vi "Osciloskop.vi"() -> ()   [LabVIEW 2026]
uses:
  <vilib>/express/express analysis/Spectral/XNode/ExpressSpectralMeasurementsBlockNode.xnode
  <vilib>/express/express analysis/Spectral/Block/exnSpectralBlock spectral measurements RMS poly.vi
  <vilib>/express/express analysis/Spectral/Block/exnSpectralBlock spectral measurements RMS DDT.vi
  <instrlib>/niScope/Controls/niScope scalar measurement.ctl
  <instrlib>/niScope/Utility/niScope Get Channel Name From String.vi
  <instrlib>/niScope/Acquire/Fetch/niScope Fetch WDT.vi
  <vilib>/express/express analysis/Spectral/Block/exnSpectralBlock spectral measurements peak poly.vi
  <vilib>/express/express analysis/Spectral/Block/exnSpectralBlock spectral measurements peak DDT.vi
  <vilib>/express/express analysis/Spectral/Block/exnSpectralBlock spectral measurements power poly.vi
  <vilib>/express/express analysis/Spectral/Block/exnSpectralBlock spectral measurements power DDT.vi
  <vilib>/express/express analysis/Spectral/Block/exnSpectralBlock spectral measurements PSD poly.vi
  <vilib>/express/express analysis/Spectral/Block/exnSpectralBlock spectral measurements PSD DDT.vi
panel:
  out "FFT":dynamicdata(graph)
  out "Waveform Graph":waveform(dbl)[](graph)
  in  "Resource name":refnum<k15> caption="Uredjaj"
  in  "Start/Pauza":bool
  in  "Simulacija":bool
  in  "Measurement 5":T1=6 caption="Measurement 4" items=["None"=4000, "Frequency"=2, "Average Frequency"=1016, "FFT Frequency"=1008, "Period"=3, "Average Period"=1015, "Rise Time"=0, "Fall Time"=1, "Rising Slew Rate"=1010, "Falling Slew Rate"=1011, "Overshoot"=18, "Preshoot"=19, "Voltage RMS"=4, "Voltage Cycle RMS"=16, "AC Estimate"=1012, "FFT Amplitude"=1009, "Voltage Average"=10, "Voltage Cycle Average"=17, "DC Estimate"=1013, "Voltage Max"=6, "Voltage Min"=7, "Voltage Peak-to-Peak"=5, "Voltage High"=8, "Voltage Low"=9, "Voltage Amplitude"=15, "Voltage Top"=1007, "Voltage Base"=1006, "Voltage Base-to-Top"=1017, "Negative Width"=11, "Positive Width"=12, "Negative Duty Cycle"=13, "Positive Duty Cycle"=14, "Integral"=1005, "Area"=1003, "Cycle Area"=1004, "Time Delay"=1014, "Phase Delay"=1018, "Low Ref Volts"=1000, "Mid Ref Volts"=1001, "High Ref Volts"=1002, "Volt. Hist. Mean"=2000, "Volt. Hist. Stdev"=2001, "Volt. Hist. Median"=2003, "Volt. Hist. Mode"=2010, "Volt. Hist. Max"=2005, "Volt. Hist. Min"=2006, "Volt. Hist. Peak-to-Peak"=2002, "Volt. Hist. Mean + Stdev"=2007, "Volt. Hist. Mean + 2 Stdev"=2008, "Volt. Hist. Mean + 3 Stdev"=2009, "Volt. Hist. Hits"=2004, "Volt. Hist. New Hits"=2011, "Time Hist. Mean"=3000, "Time Hist. Stdev"=3001, "Time Hist. Median"=3003, "Time Hist. Mode"=3010, "Time Hist. Max"=3005, "Time Hist. Min"=3006, "Time Hist. Peak-to-Peak"=3002, "Time Hist. Mean + Stdev"=3007, "Time Hist. Mean + 2 Stdev"=3008, "Time Hist. Mean + 3 Stdev"=3009, "Time Hist. Hits"=3004, "Time Hist. New Hits"=3011]
  in  "Measurement 4":T1=5 caption="Measurement 3" items=["None"=4000, "Frequency"=2, "Average Frequency"=1016, "FFT Frequency"=1008, "Period"=3, "Average Period"=1015, "Rise Time"=0, "Fall Time"=1, "Rising Slew Rate"=1010, "Falling Slew Rate"=1011, "Overshoot"=18, "Preshoot"=19, "Voltage RMS"=4, "Voltage Cycle RMS"=16, "AC Estimate"=1012, "FFT Amplitude"=1009, "Voltage Average"=10, "Voltage Cycle Average"=17, "DC Estimate"=1013, "Voltage Max"=6, "Voltage Min"=7, "Voltage Peak-to-Peak"=5, "Voltage High"=8, "Voltage Low"=9, "Voltage Amplitude"=15, "Voltage Top"=1007, "Voltage Base"=1006, "Voltage Base-to-Top"=1017, "Negative Width"=11, "Positive Width"=12, "Negative Duty Cycle"=13, "Positive Duty Cycle"=14, "Integral"=1005, "Area"=1003, "Cycle Area"=1004, "Time Delay"=1014, "Phase Delay"=1018, "Low Ref Volts"=1000, "Mid Ref Volts"=1001, "High Ref Volts"=1002, "Volt. Hist. Mean"=2000, "Volt. Hist. Stdev"=2001, "Volt. Hist. Median"=2003, "Volt. Hist. Mode"=2010, "Volt. Hist. Max"=2005, "Volt. Hist. Min"=2006, "Volt. Hist. Peak-to-Peak"=2002, "Volt. Hist. Mean + Stdev"=2007, "Volt. Hist. Mean + 2 Stdev"=2008, "Volt. Hist. Mean + 3 Stdev"=2009, "Volt. Hist. Hits"=2004, "Volt. Hist. New Hits"=2011, "Time Hist. Mean"=3000, "Time Hist. Stdev"=3001, "Time Hist. Median"=3003, "Time Hist. Mode"=3010, "Time Hist. Max"=3005, "Time Hist. Min"=3006, "Time Hist. Peak-to-Peak"=3002, "Time Hist. Mean + Stdev"=3007, "Time Hist. Mean + 2 Stdev"=3008, "Time Hist. Mean + 3 Stdev"=3009, "Time Hist. Hits"=3004, "Time Hist. New Hits"=3011]
  in  "Measurement 3":T1 caption="Measurement 2" items=["None"=4000, "Frequency"=2, "Average Frequency"=1016, "FFT Frequency"=1008, "Period"=3, "Average Period"=1015, "Rise Time"=0, "Fall Time"=1, "Rising Slew Rate"=1010, "Falling Slew Rate"=1011, "Overshoot"=18, "Preshoot"=19, "Voltage RMS"=4, "Voltage Cycle RMS"=16, "AC Estimate"=1012, "FFT Amplitude"=1009, "Voltage Average"=10, "Voltage Cycle Average"=17, "DC Estimate"=1013, "Voltage Max"=6, "Voltage Min"=7, "Voltage Peak-to-Peak"=5, "Voltage High"=8, "Voltage Low"=9, "Voltage Amplitude"=15, "Voltage Top"=1007, "Voltage Base"=1006, "Voltage Base-to-Top"=1017, "Negative Width"=11, "Positive Width"=12, "Negative Duty Cycle"=13, "Positive Duty Cycle"=14, "Integral"=1005, "Area"=1003, "Cycle Area"=1004, "Time Delay"=1014, "Phase Delay"=1018, "Low Ref Volts"=1000, "Mid Ref Volts"=1001, "High Ref Volts"=1002, "Volt. Hist. Mean"=2000, "Volt. Hist. Stdev"=2001, "Volt. Hist. Median"=2003, "Volt. Hist. Mode"=2010, "Volt. Hist. Max"=2005, "Volt. Hist. Min"=2006, "Volt. Hist. Peak-to-Peak"=2002, "Volt. Hist. Mean + Stdev"=2007, "Volt. Hist. Mean + 2 Stdev"=2008, "Volt. Hist. Mean + 3 Stdev"=2009, "Volt. Hist. Hits"=2004, "Volt. Hist. New Hits"=2011, "Time Hist. Mean"=3000, "Time Hist. Stdev"=3001, "Time Hist. Median"=3003, "Time Hist. Mode"=3010, "Time Hist. Max"=3005, "Time Hist. Min"=3006, "Time Hist. Peak-to-Peak"=3002, "Time Hist. Mean + Stdev"=3007, "Time Hist. Mean + 2 Stdev"=3008, "Time Hist. Mean + 3 Stdev"=3009, "Time Hist. Hits"=3004, "Time Hist. New Hits"=3011]
  in  "Measurement 2":T1=2 caption="Measurement 1" items=["None"=4000, "Frequency"=2, "Average Frequency"=1016, "FFT Frequency"=1008, "Period"=3, "Average Period"=1015, "Rise Time"=0, "Fall Time"=1, "Rising Slew Rate"=1010, "Falling Slew Rate"=1011, "Overshoot"=18, "Preshoot"=19, "Voltage RMS"=4, "Voltage Cycle RMS"=16, "AC Estimate"=1012, "FFT Amplitude"=1009, "Voltage Average"=10, "Voltage Cycle Average"=17, "DC Estimate"=1013, "Voltage Max"=6, "Voltage Min"=7, "Voltage Peak-to-Peak"=5, "Voltage High"=8, "Voltage Low"=9, "Voltage Amplitude"=15, "Voltage Top"=1007, "Voltage Base"=1006, "Voltage Base-to-Top"=1017, "Negative Width"=11, "Positive Width"=12, "Negative Duty Cycle"=13, "Positive Duty Cycle"=14, "Integral"=1005, "Area"=1003, "Cycle Area"=1004, "Time Delay"=1014, "Phase Delay"=1018, "Low Ref Volts"=1000, "Mid Ref Volts"=1001, "High Ref Volts"=1002, "Volt. Hist. Mean"=2000, "Volt. Hist. Stdev"=2001, "Volt. Hist. Median"=2003, "Volt. Hist. Mode"=2010, "Volt. Hist. Max"=2005, "Volt. Hist. Min"=2006, "Volt. Hist. Peak-to-Peak"=2002, "Volt. Hist. Mean + Stdev"=2007, "Volt. Hist. Mean + 2 Stdev"=2008, "Volt. Hist. Mean + 3 Stdev"=2009, "Volt. Hist. Hits"=2004, "Volt. Hist. New Hits"=2011, "Time Hist. Mean"=3000, "Time Hist. Stdev"=3001, "Time Hist. Median"=3003, "Time Hist. Mode"=3010, "Time Hist. Max"=3005, "Time Hist. Min"=3006, "Time Hist. Peak-to-Peak"=3002, "Time Hist. Mean + Stdev"=3007, "Time Hist. Mean + 2 Stdev"=3008, "Time Hist. Mean + 3 Stdev"=3009, "Time Hist. Hits"=3004, "Time Hist. New Hits"=3011]
  in  "Velicina":T2(ring)
  in  "Left/Right":dbl(knob) scale=-100.0..100.0
  in  "Amplituda":dbl=1.0 min=1.0 max=1000.0
  in  "Prosek":enum16{"None", "RMS", "Peak hold"}(ring)
  in  "Prozor":T3(ring)
  in  "FFT":bool
  in  "Gornji Cut-Off":dbl=10.0 caption="Lower Cut-Off"
  in  "Zoom H":dbl(knob)=1.0 scale=0.0..10.0
  in  "Zoom V":dbl(knob)=1.0 scale=0.0..10.0
  in  "Filter":T4(ring)
  in  "Donji Cut-Off":dbl=0.5 caption="Lower Cut-Off"
  in  "Down/Up":dbl(knob) scale=-100.0..100.0
  out "M5":dbl caption="Result  4" format="%.2f"
  out "M4":dbl caption="Result  3" format="%.2f"
  out "M3":dbl caption="Result  2" format="%.2f"
  out "M2":dbl caption="Result 1" format="%.2f"
  in  "Channel/s":enum16{""}(ring)
  in  "?":bool
  # "Vertical"
  # "Horizontal"
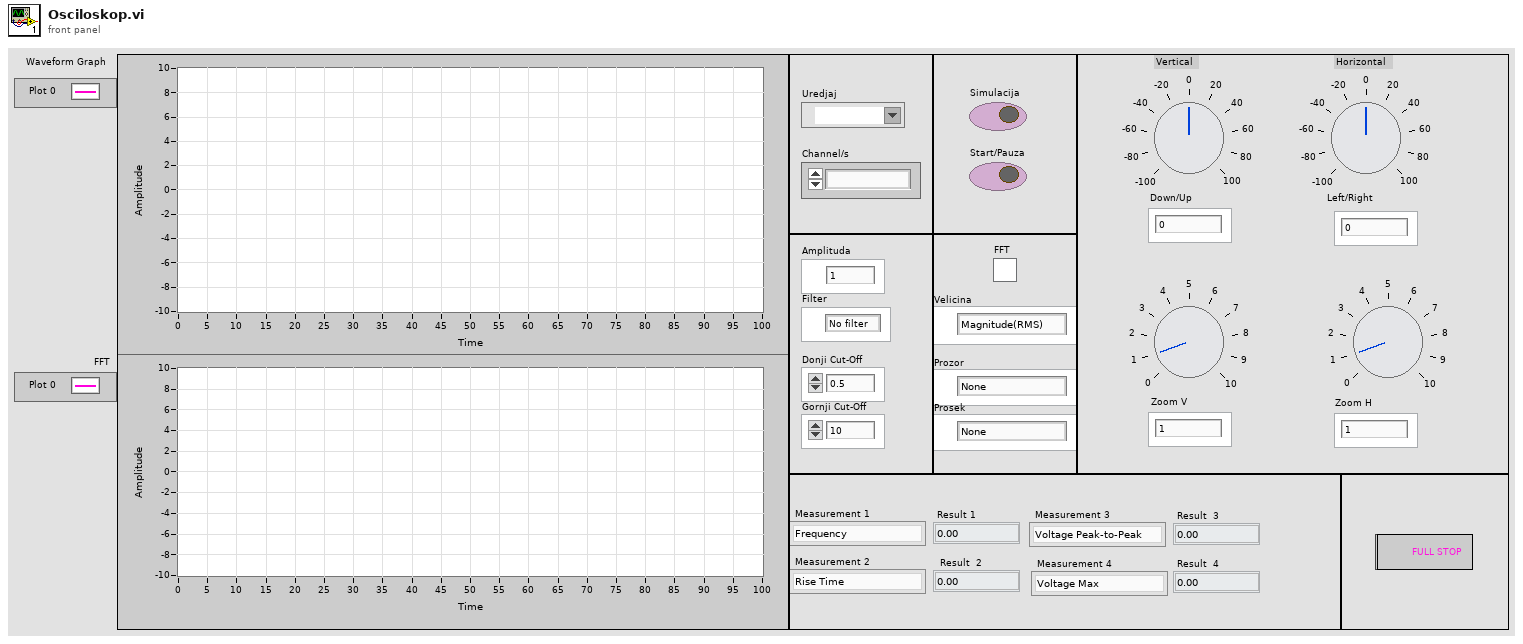
[diagram p1: front panel]
types:
  T1 = typedef "niScope scalar measurement.ctl" = i32
  T2 = enum16{"Magnitude(RMS)", "Magnitude(Peak)", "Power spectrum", "Power spectral density"}
  T3 = enum16{"None", "Hanning", "Hamming", "Blackman-Harris", "Exact Blackman", "Blackman", "Flat Top", "4 Term B-Harris", "7 Term B-Harris", "Low Sidelobe"}
  T4 = enum16{"No filter", "Low pass", "High pass", "Band pass", "Band reject", "Smoothing"}
  T5 = cluster{"averaging mode":u16, "weighting mode":u16, "number of averages":u32}
  T6 = cluster{"dB On (F)":bool, "unwrap phase (F)":bool, "convert to degree (F)":bool}
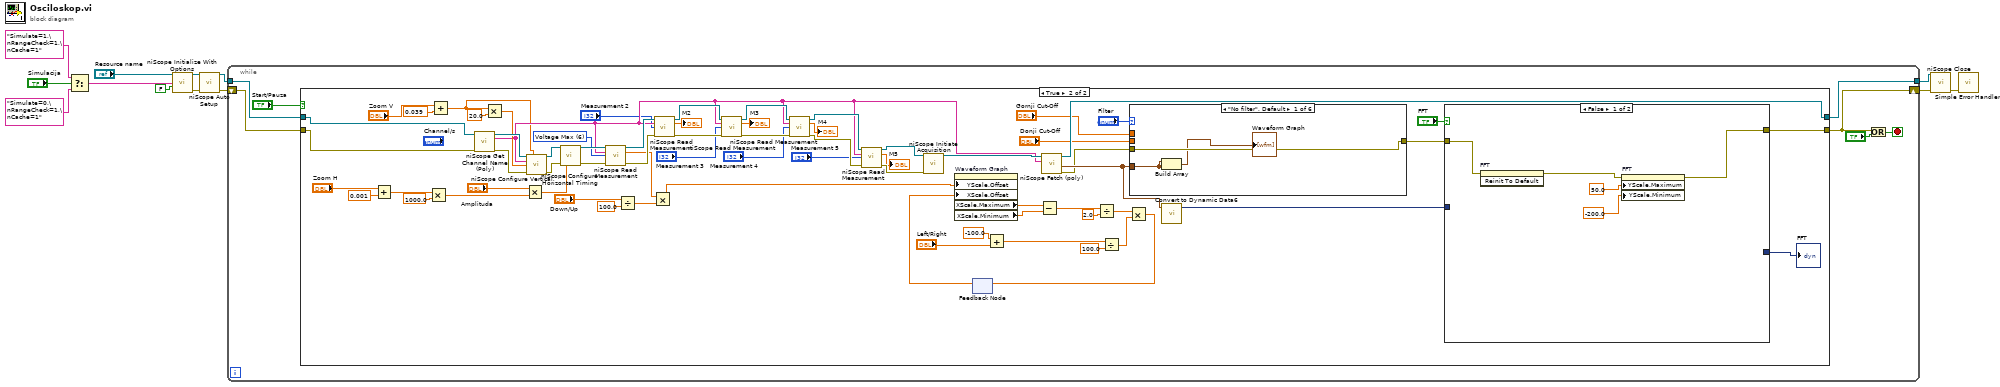
[diagram p0: block diagram]
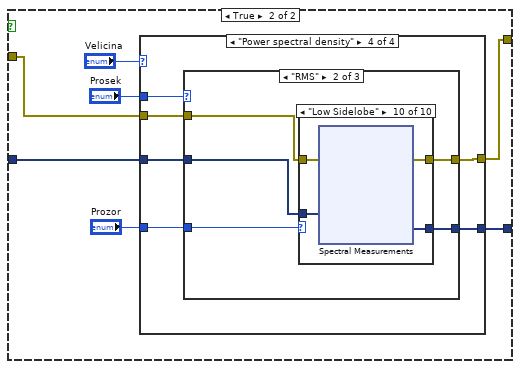
[diagram p3: hidden frame]
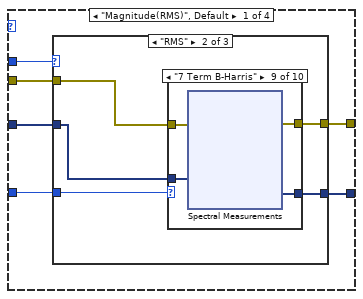
[diagram p4: hidden frame]
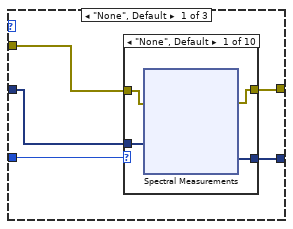
[diagram p5: hidden frame]
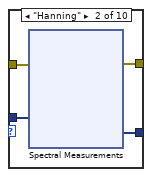
[diagram p6: hidden frame]
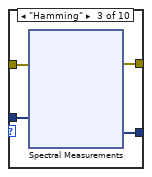
[diagram p7: hidden frame]
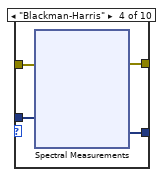
[diagram p8: hidden frame]
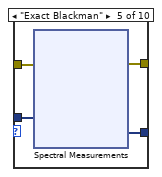
[diagram p9: hidden frame]
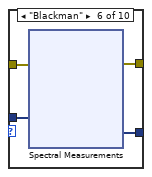
[diagram p10: hidden frame]
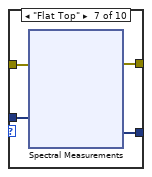
[diagram p11: hidden frame]
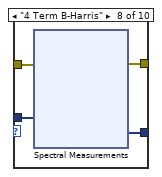
[diagram p12: hidden frame]
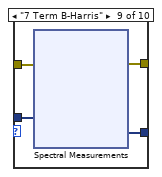
[diagram p13: hidden frame]
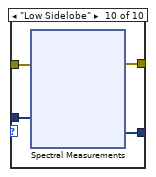
[diagram p14: hidden frame]
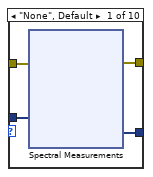
[diagram p15: hidden frame]
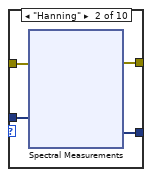
[diagram p16: hidden frame]
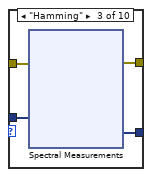
[diagram p17: hidden frame]
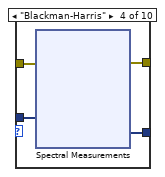
[diagram p18: hidden frame]
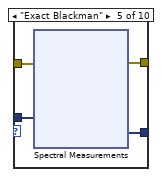
[diagram p19: hidden frame]
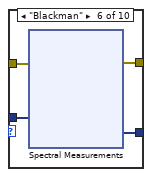
[diagram p20: hidden frame]
diagram:
  n1 = Select(t="Simulate=1,\nRangeCheck=1,\nCache=1" ("option string"), s="Simulacija", f="Simulate=0,\nRangeCheck=1,\nCache=1" ("option string")) -> (s? t:f=w9:string)
  n2 = call <instrlib>:"niScope Initialize With Options.vi"("resource name"="Resource name", "option string"=w9, "reset device"=FALSE) -> ("instrument handle"=w7:refnum<k15>, "error out"=w8:errorcluster)  [unwired: 11 in]
  n3 = call <instrlib>:"niScope Auto Setup.vi"("instrument handle"=w7, "error in"=w8) -> ("instrument handle out"=w6:refnum<k15>, "error out"=w4:errorcluster)  [unwired: 12 in]
  n4 = while {
    tunnel: w6 -> [w18]
    shift-right: [w15] -> w5
    shift-left: w4 -> [w17]
    tunnel: [w16] -> w3
    stop <- w19 stop-if-true
    n5 = case shown="True" "Start/Pauza" {
      tunnel: [w21 w89] -> w16
      tunnel: w17 -> [w22 w61]
      tunnel: w18 -> [w21 w60]
      tunnel: [w22 w59] -> w15
      frame False {
      }
      frame True {
        w31 = T1 6 items=["None"=4000, "Frequency"=2, "Average Frequency"=1016, "FFT Frequency"=1008, "Period"=3, "Average Period"=1015, "Rise Time"=0, "Fall Time"=1, "Rising Slew Rate"=1010, "Falling Slew Rate"=1011, "Overshoot"=18, "Preshoot"=19, "Voltage RMS"=4, "Voltage Cycle RMS"=16, "AC Estimate"=1012, "FFT Amplitude"=1009, "Voltage Average"=10, "Voltage Cycle Average"=17, "DC Estimate"=1013, "Voltage Max"=6, "Voltage Min"=7, "Voltage Peak-to-Peak"=5, "Voltage High"=8, "Voltage Low"=9, "Voltage Amplitude"=15, "Voltage Top"=1007, "Voltage Base"=1006, "Voltage Base-to-Top"=1017, "Negative Width"=11, "Positive Width"=12, "Negative Duty Cycle"=13, "Positive Duty Cycle"=14, "Integral"=1005, "Area"=1003, "Cycle Area"=1004, "Time Delay"=1014, "Phase Delay"=1018, "Low Ref Volts"=1000, "Mid Ref Volts"=1001, "High Ref Volts"=1002, "Volt. Hist. Mean"=2000, "Volt. Hist. Stdev"=2001, "Volt. Hist. Median"=2003, "Volt. Hist. Mode"=2010, "Volt. Hist. Max"=2005, "Volt. Hist. Min"=2006, "Volt. Hist. Peak-to-Peak"=2002, "Volt. Hist. Mean + Stdev"=2007, "Volt. Hist. Mean + 2 Stdev"=2008, "Volt. Hist. Mean + 3 Stdev"=2009, "Volt. Hist. Hits"=2004, "Volt. Hist. New Hits"=2011, "Time Hist. Mean"=3000, "Time Hist. Stdev"=3001, "Time Hist. Median"=3003, "Time Hist. Mode"=3010, "Time Hist. Max"=3005, "Time Hist. Min"=3006, "Time Hist. Peak-to-Peak"=3002, "Time Hist. Mean + Stdev"=3007, "Time Hist. Mean + 2 Stdev"=3008, "Time Hist. Mean + 3 Stdev"=3009, "Time Hist. Hits"=3004, "Time Hist. New Hits"=3011] ("scalar measurement")
        n6 = Add(x="Zoom H", y=0.001) -> (x+y=w47:dbl)
        n7 = Multiply(x=w47, y=1000.0 ("x")) -> (x*y=w46:dbl)
        n8 = Add(x="Zoom V", y=0.039) -> (x+y=w28:dbl)
        n9 = call-poly <instrlib>:"niScope Get Channel Name (Poly).vi"("instrument handle"=w60, "error in"=w61) -> ("instrument handle out"=w91:refnum<k15>, "channel name"=w56:string, "error out"=w90:errorcluster)  [unwired: 11 in]
        n10 = Multiply(x=w28, y=20.0) -> (x*y=w83:dbl)
        n11 = Multiply(x="Amplituda", y=w46) -> (x*y=w82:dbl)
        n12 = call <instrlib>:"niScope Configure Vertical.vi"("instrument handle"=w91, "probe attenuation"=w28, "channels"=w56, "vertical range"=w83, "error in"=w90) -> ("instrument handle out"=w29:refnum<k15>, "error out"=w30:errorcluster)  [unwired: 9 in]
        n13 = call <instrlib>:"niScope Configure Horizontal Timing.vi"("instrument handle"=w29, "error in"=w30, "min record length"=w82) -> ("instrument handle out"=w78:refnum<k15>, "error out"=w79:errorcluster)  [unwired: 11 in]
        n14 = call <instrlib>:"niScope Read Measurement.vi"("instrument handle"=w78, "channels"=w56, "scalar measurement"=w31, "error in"=w79) -> ("instrument handle out"=w71:refnum<k15>, "result"=w55:dbl, "error out"=w66:errorcluster)  [unwired: 9 in]
        n15 = Divide(x="Down/Up", y=100.0) -> (x/y=w41:dbl)
        n16 = Multiply(x=w55, y=w41) -> (x*y=w26:dbl)
        n17 = call <instrlib>:"niScope Read Measurement.vi"("instrument handle"=w71, "channels"=w56, "scalar measurement"="Measurement 2", "error in"=w66) -> ("instrument handle out"=w70:refnum<k15>, "result"=→"M2":dbl, "error out"=w65:errorcluster)  [unwired: 9 in]
        n18 = call <instrlib>:"niScope Read Measurement.vi"("instrument handle"=w70, "channels"=w56, "scalar measurement"="Measurement 3", "error in"=w65) -> ("instrument handle out"=w69:refnum<k15>, "result"=→"M3":dbl, "error out"=w64:errorcluster)  [unwired: 9 in]
        n19 = call <instrlib>:"niScope Read Measurement.vi"("instrument handle"=w69, "channels"=w56, "scalar measurement"="Measurement 4", "error in"=w64) -> ("instrument handle out"=w68:refnum<k15>, "result"=→"M4":dbl, "error out"=w63:errorcluster)  [unwired: 9 in]
        n20 = call <instrlib>:"niScope Read Measurement.vi"("instrument handle"=w68, "channels"=w56, "scalar measurement"="Measurement 5", "error in"=w63) -> ("instrument handle out"=w67:refnum<k15>, "result"=→"M5":dbl, "error out"=w62:errorcluster)  [unwired: 9 in]
        n21 = call <instrlib>:"niScope Initiate Acquisition.vi"("instrument handle"=w67, "error in"=w62) -> ("instrument handle out"=w80:refnum<k15>)  [unwired: 12 in, 1 out]
        n22 = feedback #1() -> (w25:dbl)  [unwired: 1 in]
        n23 = property on="Waveform Graph" class="WFGraph (strict)"("YScale.Offset"=w26, "XScale.Offset"=w25) -> ("XScale.Maximum"=w24:dbl, "XScale.Minimum"=w23:dbl)  [unwired: 2 in, 2 out]
        n24 = Add(x=-100.0, y="Left/Right") -> (x+y=w38:dbl)
        n25 = Subtract(x=w24, y=w23) -> (x-y=w77:dbl)
        n26 = call-poly <instrlib>:"niScope Fetch (poly).vi"("channels"=w56, "instrument handle"=w80) -> ("error out"=w32:errorcluster, "wfm"=w33:waveform(dbl), "instrument handle out"=w89:refnum<k15>)  [unwired: 6 in, 1 out]
        n27 = Divide(x=w77, y=2.0) -> (x/y=w75:dbl)
        n28 = Divide(x=w38, y=100.0) -> (x/y=w37:dbl)
        n29 = Multiply(x=w75, y=w37) -> (x*y=w74:dbl)
        n30 = feedback-in #1(w74) -> ()
        n31 = case shown="\"No filter\", Default" "Filter" {
          tunnel: "Donji Cut-Off" -> [_ w1897 w1905 w1915 w1924 _]
          tunnel: w33 -> [w1890 w1894 w1902 w1911 w1920 w1929]
          tunnel: "Gornji Cut-Off" -> [_ _ _ w1909 w1918 _]
          tunnel: w32 -> [w1889 w1892 w1900 w1907 w1917 w1925]
          tunnel: [w1889 w1891 w1899 w1908 w1916 w1926] -> w58
          frame "No filter", Default {
            n32 = Build Array(w1890, w1890) -> (→"Waveform Graph":waveform(dbl)[])
          }
          frame "Low pass" {
            n33 = call "Convert to Dynamic Data2"("Waveform"=w1894) -> ("Dynamic Data Type"=w1896:dynamicdata)  [unwired: 3 in]
            n34 = call "Filter2"("error in (no error)"=w1892, "Lower Cut-Off"=w1897, "Signal"=w1896) -> ("error out"=w1891:errorcluster, "Filtered Signal"=w1898:dynamicdata)  [unwired: 7 in]
            n35 = call "Convert from Dynamic Data2"("Dynamic Data Type"=w1898) -> ("Waveform"=w1895:waveform(dbl))  [unwired: 3 in]
            n36 = Build Array(w1895, w1894) -> (w1893:waveform(dbl)[])
            n37 = local write "Waveform Graph"(w1893) -> ()
          }
          frame "High pass" {
            n38 = call "Convert to Dynamic Data3"("Waveform"=w1902) -> ("Dynamic Data Type"=w1904:dynamicdata)  [unwired: 3 in]
            n39 = call "Filter3"("error in (no error)"=w1900, "Lower Cut-Off"=w1905, "Signal"=w1904) -> ("error out"=w1899:errorcluster, "Filtered Signal"=w1906:dynamicdata)  [unwired: 7 in]
            n40 = call "Convert from Dynamic Data3"("Dynamic Data Type"=w1906) -> ("Waveform"=w1903:waveform(dbl))  [unwired: 3 in]
            n41 = Build Array(w1903, w1902) -> (w1901:waveform(dbl)[])
            n42 = local write "Waveform Graph"(w1901) -> ()
          }
          frame "Band pass" {
            n43 = call "Convert to Dynamic Data4"("Waveform"=w1911) -> ("Dynamic Data Type"=w1914:dynamicdata)  [unwired: 3 in]
            n44 = call "Filter4"("error in (no error)"=w1907, "Lower Cut-Off"=w1915, "Upper Cut-Off"=w1909, "Signal"=w1914) -> ("error out"=w1908:errorcluster, "Filtered Signal"=w1913:dynamicdata)  [unwired: 6 in]
            n45 = call "Convert from Dynamic Data4"("Dynamic Data Type"=w1913, "Channel"=w1913) -> ("Waveform"=w1912:waveform(dbl))  [unwired: 2 in]
            n46 = Build Array(w1912, w1911) -> (w1910:waveform(dbl)[])
            n47 = local write "Waveform Graph"(w1910) -> ()
          }
          frame "Band reject" {
            n48 = call "Convert to Dynamic Data"("Waveform"=w1920) -> ("Dynamic Data Type"=w1923:dynamicdata)  [unwired: 3 in]
            n49 = call "Filter"("error in (no error)"=w1917, "Lower Cut-Off"=w1924, "Upper Cut-Off"=w1918, "Signal"=w1923) -> ("error out"=w1916:errorcluster, "Filtered Signal"=w1922:dynamicdata)  [unwired: 6 in]
            n50 = call "Convert from Dynamic Data"("Dynamic Data Type"=w1922, "Channel"=w1922) -> ("Waveform"=w1921:waveform(dbl))  [unwired: 2 in]
            n51 = Build Array(w1921, w1920) -> (w1919:waveform(dbl)[])
            n52 = local write "Waveform Graph"(w1919) -> ()
          }
          frame "Smoothing" {
            n53 = call "Convert to Dynamic Data5"("Waveform"=w1929) -> ("Dynamic Data Type"=w1931:dynamicdata)  [unwired: 3 in]
            n54 = call "Filter5"("error in (no error)"=w1925, "Signal"=w1931) -> ("error out"=w1926:errorcluster, "Filtered Signal"=w1930:dynamicdata)  [unwired: 8 in]
            n55 = call "Convert from Dynamic Data5"("Dynamic Data Type"=w1930, "Channel"=w1930) -> ("Waveform"=w1927:waveform(dbl))  [unwired: 2 in]
            n56 = Build Array(w1927, w1927) -> (w1928:waveform(dbl)[])
            n57 = local write "Waveform Graph"(w1928) -> ()
          }
        }
        n58 = call "Convert to Dynamic Data6"("Waveform"=w33) -> ("Dynamic Data Type"=w84:dynamicdata)  [unwired: 3 in]
        n59 = case shown="False" "FFT" {
          tunnel: w58 -> [w96 w101]
          tunnel: [w92 w99] -> w59
          tunnel: w84 -> [_ w100]
          tunnel: [_ w97] -> w27
          frame False {
            n60 = invoke on="FFT" class="WFGraph (strict)" method="Reinit To Default"(error in=w96) -> (error out=w95:errorcluster)  [unwired: 2 in, 2 out]
            n61 = property on="FFT" class="WFGraph (strict)"(error in=w95, "YScale.Maximum"=50.0 ("Y Scale.Range:Maximum"), "YScale.Minimum"=-200.0 ("Y Scale.Range:Minimum")) -> (error out=w92:errorcluster)  [unwired: 1 in, 1 out]
          }
          frame True {
            n62 = case shown="\"Power spectral density\"" "Velicina" {
              tunnel: "Prosek" -> [w109 w570 w1031 w1462]
              tunnel: "Prozor" -> [w108 w569 w1030 w1461]
              tunnel: w101 -> [w107 w568 w1029 w1460]
              tunnel: w100 -> [w106 w567 w1028 w1459]
              tunnel: [w105 w566 w1027 w1458] -> w99
              tunnel: [w104 w565 w1026 w1457] -> w97
              frame "Magnitude(RMS)", Default {
                n63 = case shown="\"RMS\"" w109 {
                  tunnel: w108 -> [w114 w259 w414]
                  tunnel: w107 -> [w113 w258 w413]
                  tunnel: w106 -> [w112 w257 w412]
                  tunnel: [w111 w256 w411] -> w105
                  tunnel: [w110 w255 w410] -> w104
                  frame "None", Default {
                    n64 = case shown="\"None\", Default" w114 {
                      tunnel: w113 -> [w118 w132 w146 w160 w174 w188 w202 w216 w230 w244]
                      tunnel: w112 -> [w117 w131 w145 w159 w173 w187 w201 w215 w229 w243]
                      tunnel: [w116 w130 w144 w158 w172 w186 w200 w214 w228 w242] -> w111
                      tunnel: [w115 w129 w143 w157 w171 w185 w199 w213 w227 w241] -> w110
                      frame "None", Default {
                        n65 = xnode "Spectral Measurements"("Signals"=w117, "error in (no error)"=w118) -> ("FFT - (RMS)"=w115:dynamicdata, "error out"=w116:errorcluster)  [unwired: 1 out]
                      }
                      frame "Hanning" {
                        n66 = xnode "Spectral Measurements"("Signals"=w131, "error in (no error)"=w132) -> ("FFT - (RMS)"=w129:dynamicdata, "error out"=w130:errorcluster)  [unwired: 1 out]
                      }
                      frame "Hamming" {
                        n67 = xnode "Spectral Measurements"("Signals"=w145, "error in (no error)"=w146) -> ("FFT - (RMS)"=w143:dynamicdata, "error out"=w144:errorcluster)  [unwired: 1 out]
                      }
                      frame "Blackman-Harris" {
                        n68 = xnode "Spectral Measurements"("Signals"=w159, "error in (no error)"=w160) -> ("FFT - (RMS)"=w157:dynamicdata, "error out"=w158:errorcluster)  [unwired: 1 out]
                      }
                      frame "Exact Blackman" {
                        n69 = xnode "Spectral Measurements"("Signals"=w173, "error in (no error)"=w174) -> ("FFT - (RMS)"=w171:dynamicdata, "error out"=w172:errorcluster)  [unwired: 1 out]
                      }
                      frame "Blackman" {
                        n70 = xnode "Spectral Measurements"("Signals"=w187, "error in (no error)"=w188) -> ("FFT - (RMS)"=w185:dynamicdata, "error out"=w186:errorcluster)  [unwired: 1 out]
                      }
                      frame "Flat Top" {
                        n71 = xnode "Spectral Measurements"("Signals"=w201, "error in (no error)"=w202) -> ("FFT - (RMS)"=w199:dynamicdata, "error out"=w200:errorcluster)  [unwired: 1 out]
                      }
                      frame "4 Term B-Harris" {
                        n72 = xnode "Spectral Measurements"("Signals"=w215, "error in (no error)"=w216) -> ("FFT - (RMS)"=w213:dynamicdata, "error out"=w214:errorcluster)  [unwired: 1 out]
                      }
                      frame "7 Term B-Harris" {
                        n73 = xnode "Spectral Measurements"("Signals"=w229, "error in (no error)"=w230) -> ("FFT - (RMS)"=w227:dynamicdata, "error out"=w228:errorcluster)  [unwired: 1 out]
                      }
                      frame "Low Sidelobe" {
                        n74 = xnode "Spectral Measurements"("Signals"=w243, "error in (no error)"=w244) -> ("FFT - (RMS)"=w241:dynamicdata, "error out"=w242:errorcluster)  [unwired: 1 out]
                      }
                    }
                  }
                  frame "RMS" {
                    n75 = case shown="\"7 Term B-Harris\"" w259 {
                      tunnel: w258 -> [w263 w278 w293 w308 w323 w338 w353 w368 w383 w398]
                      tunnel: w257 -> [w262 w277 w292 w307 w322 w337 w352 w367 w382 w397]
                      tunnel: [w261 w276 w291 w306 w321 w336 w351 w366 w381 w396] -> w256
                      tunnel: [w260 w275 w290 w305 w320 w335 w350 w365 w380 w395] -> w255
                      frame "None", Default {
                        n76 = xnode "Spectral Measurements"("Signals"=w262, "error in (no error)"=w263) -> ("FFT - (RMS)"=w260:dynamicdata, "error out"=w261:errorcluster)  [unwired: 1 in, 2 out]
                      }
                      frame "Hanning" {
                        n77 = xnode "Spectral Measurements"("Signals"=w277, "error in (no error)"=w278) -> ("FFT - (RMS)"=w275:dynamicdata, "error out"=w276:errorcluster)  [unwired: 1 in, 2 out]
                      }
                      frame "Hamming" {
                        n78 = xnode "Spectral Measurements"("Signals"=w292, "error in (no error)"=w293) -> ("FFT - (RMS)"=w290:dynamicdata, "error out"=w291:errorcluster)  [unwired: 1 in, 2 out]
                      }
                      frame "Blackman-Harris" {
                        n79 = xnode "Spectral Measurements"("Signals"=w307, "error in (no error)"=w308) -> ("FFT - (RMS)"=w305:dynamicdata, "error out"=w306:errorcluster)  [unwired: 1 in, 2 out]
                      }
                      frame "Exact Blackman" {
                        n80 = xnode "Spectral Measurements"("Signals"=w322, "error in (no error)"=w323) -> ("FFT - (RMS)"=w320:dynamicdata, "error out"=w321:errorcluster)  [unwired: 1 in, 2 out]
                      }
                      frame "Blackman" {
                        n81 = xnode "Spectral Measurements"("Signals"=w337, "error in (no error)"=w338) -> ("FFT - (RMS)"=w335:dynamicdata, "error out"=w336:errorcluster)  [unwired: 1 in, 2 out]
                      }
                      frame "Flat Top" {
                        n82 = xnode "Spectral Measurements"("Signals"=w352, "error in (no error)"=w353) -> ("FFT - (RMS)"=w350:dynamicdata, "error out"=w351:errorcluster)  [unwired: 1 in, 2 out]
                      }
                      frame "4 Term B-Harris" {
                        n83 = xnode "Spectral Measurements"("Signals"=w367, "error in (no error)"=w368) -> ("FFT - (RMS)"=w365:dynamicdata, "error out"=w366:errorcluster)  [unwired: 1 in, 2 out]
                      }
                      frame "7 Term B-Harris" {
                        n84 = xnode "Spectral Measurements"("Signals"=w382, "error in (no error)"=w383) -> ("FFT - (RMS)"=w380:dynamicdata, "error out"=w381:errorcluster)  [unwired: 1 in, 2 out]
                      }
                      frame "Low Sidelobe" {
                        n85 = xnode "Spectral Measurements"("Signals"=w397, "error in (no error)"=w398) -> ("FFT - (RMS)"=w395:dynamicdata, "error out"=w396:errorcluster)  [unwired: 1 in, 2 out]
                      }
                    }
                  }
                  frame "Peak hold" {
                    n86 = case shown="\"Low Sidelobe\"" w414 {
                      tunnel: w413 -> [w418 w433 w448 w463 w478 w493 w508 w523 w538 w553]
                      tunnel: w412 -> [w417 w432 w447 w462 w477 w492 w507 w522 w537 w552]
                      tunnel: [w416 w431 w446 w461 w476 w491 w506 w521 w536 w551] -> w411
                      tunnel: [w415 w430 w445 w460 w475 w490 w505 w520 w535 w550] -> w410
                      frame "None", Default {
                        n87 = xnode "Spectral Measurements"("Signals"=w417, "error in (no error)"=w418) -> ("FFT - (RMS)"=w415:dynamicdata, "error out"=w416:errorcluster)  [unwired: 1 in, 2 out]
                      }
                      frame "Hanning" {
                        n88 = xnode "Spectral Measurements"("Signals"=w432, "error in (no error)"=w433) -> ("FFT - (RMS)"=w430:dynamicdata, "error out"=w431:errorcluster)  [unwired: 1 in, 2 out]
                      }
                      frame "Hamming" {
                        n89 = xnode "Spectral Measurements"("Signals"=w447, "error in (no error)"=w448) -> ("FFT - (RMS)"=w445:dynamicdata, "error out"=w446:errorcluster)  [unwired: 1 in, 2 out]
                      }
                      frame "Blackman-Harris" {
                        n90 = xnode "Spectral Measurements"("Signals"=w462, "error in (no error)"=w463) -> ("FFT - (RMS)"=w460:dynamicdata, "error out"=w461:errorcluster)  [unwired: 1 in, 2 out]
                      }
                      frame "Exact Blackman" {
                        n91 = xnode "Spectral Measurements"("Signals"=w477, "error in (no error)"=w478) -> ("FFT - (RMS)"=w475:dynamicdata, "error out"=w476:errorcluster)  [unwired: 1 in, 2 out]
                      }
                      frame "Blackman" {
                        n92 = xnode "Spectral Measurements"("Signals"=w492, "error in (no error)"=w493) -> ("FFT - (RMS)"=w490:dynamicdata, "error out"=w491:errorcluster)  [unwired: 1 in, 2 out]
                      }
                      frame "Flat Top" {
                        n93 = xnode "Spectral Measurements"("Signals"=w507, "error in (no error)"=w508) -> ("FFT - (RMS)"=w505:dynamicdata, "error out"=w506:errorcluster)  [unwired: 1 in, 2 out]
                      }
                      frame "4 Term B-Harris" {
                        n94 = xnode "Spectral Measurements"("Signals"=w522, "error in (no error)"=w523) -> ("FFT - (RMS)"=w520:dynamicdata, "error out"=w521:errorcluster)  [unwired: 1 in, 2 out]
                      }
                      frame "7 Term B-Harris" {
                        n95 = xnode "Spectral Measurements"("Signals"=w537, "error in (no error)"=w538) -> ("FFT - (RMS)"=w535:dynamicdata, "error out"=w536:errorcluster)  [unwired: 1 in, 2 out]
                      }
                      frame "Low Sidelobe" {
                        n96 = xnode "Spectral Measurements"("Signals"=w552, "error in (no error)"=w553) -> ("FFT - (RMS)"=w550:dynamicdata, "error out"=w551:errorcluster)  [unwired: 1 in, 2 out]
                      }
                    }
                  }
                }
              }
              frame "Magnitude(Peak)" {
                n97 = case shown="\"Peak hold\"" w570 {
                  tunnel: w569 -> [w575 w720 w875]
                  tunnel: w568 -> [w574 w719 w874]
                  tunnel: w567 -> [w573 w718 w873]
                  tunnel: [w572 w717 w872] -> w566
                  tunnel: [w571 w716 w871] -> w565
                  frame "None", Default {
                    n98 = case shown="\"Low Sidelobe\"" w575 {
                      tunnel: w574 -> [w579 w593 w607 w621 w635 w649 w663 w677 w691 w705]
                      tunnel: w573 -> [w578 w592 w606 w620 w634 w648 w662 w676 w690 w704]
                      tunnel: [w577 w591 w605 w619 w633 w647 w661 w675 w689 w703] -> w572
                      tunnel: [w576 w590 w604 w618 w632 w646 w660 w674 w688 w702] -> w571
                      frame "None", Default {
                        n99 = xnode "Spectral Measurements"("Signals"=w578, "error in (no error)"=w579) -> ("FFT - (Peak)"=w576:dynamicdata, "error out"=w577:errorcluster)  [unwired: 1 out]
                      }
                      frame "Hanning" {
                        n100 = xnode "Spectral Measurements"("Signals"=w592, "error in (no error)"=w593) -> ("FFT - (Peak)"=w590:dynamicdata, "error out"=w591:errorcluster)  [unwired: 1 out]
                      }
                      frame "Hamming" {
                        n101 = xnode "Spectral Measurements"("Signals"=w606, "error in (no error)"=w607) -> ("FFT - (Peak)"=w604:dynamicdata, "error out"=w605:errorcluster)  [unwired: 1 out]
                      }
                      frame "Blackman-Harris" {
                        n102 = xnode "Spectral Measurements"("Signals"=w620, "error in (no error)"=w621) -> ("FFT - (Peak)"=w618:dynamicdata, "error out"=w619:errorcluster)  [unwired: 1 out]
                      }
                      frame "Exact Blackman" {
                        n103 = xnode "Spectral Measurements"("Signals"=w634, "error in (no error)"=w635) -> ("FFT - (Peak)"=w632:dynamicdata, "error out"=w633:errorcluster)  [unwired: 1 out]
                      }
                      frame "Blackman" {
                        n104 = xnode "Spectral Measurements"("Signals"=w648, "error in (no error)"=w649) -> ("FFT - (Peak)"=w646:dynamicdata, "error out"=w647:errorcluster)  [unwired: 1 out]
                      }
                      frame "Flat Top" {
                        n105 = xnode "Spectral Measurements"("Signals"=w662, "error in (no error)"=w663) -> ("FFT - (Peak)"=w660:dynamicdata, "error out"=w661:errorcluster)  [unwired: 1 out]
                      }
                      frame "4 Term B-Harris" {
                        n106 = xnode "Spectral Measurements"("Signals"=w676, "error in (no error)"=w677) -> ("FFT - (Peak)"=w674:dynamicdata, "error out"=w675:errorcluster)  [unwired: 1 out]
                      }
                      frame "7 Term B-Harris" {
                        n107 = xnode "Spectral Measurements"("Signals"=w690, "error in (no error)"=w691) -> ("FFT - (Peak)"=w688:dynamicdata, "error out"=w689:errorcluster)  [unwired: 1 out]
                      }
                      frame "Low Sidelobe" {
                        n108 = xnode "Spectral Measurements"("Signals"=w704, "error in (no error)"=w705) -> ("FFT - (Peak)"=w702:dynamicdata, "error out"=w703:errorcluster)  [unwired: 1 out]
                      }
                    }
                  }
                  frame "RMS" {
                    n109 = case shown="\"Low Sidelobe\"" w720 {
                      tunnel: w719 -> [w724 w739 w754 w769 w784 w799 w814 w829 w844 w859]
                      tunnel: w718 -> [w723 w738 w753 w768 w783 w798 w813 w828 w843 w858]
                      tunnel: [w722 w737 w752 w767 w782 w797 w812 w827 w842 w857] -> w717
                      tunnel: [w721 w736 w751 w766 w781 w796 w811 w826 w841 w856] -> w716
                      frame "None", Default {
                        n110 = xnode "Spectral Measurements"("Signals"=w723, "error in (no error)"=w724) -> ("FFT - (Peak)"=w721:dynamicdata, "error out"=w722:errorcluster)  [unwired: 1 in, 2 out]
                      }
                      frame "Hanning" {
                        n111 = xnode "Spectral Measurements"("Signals"=w738, "error in (no error)"=w739) -> ("FFT - (Peak)"=w736:dynamicdata, "error out"=w737:errorcluster)  [unwired: 1 in, 2 out]
                      }
                      frame "Hamming" {
                        n112 = xnode "Spectral Measurements"("Signals"=w753, "error in (no error)"=w754) -> ("FFT - (Peak)"=w751:dynamicdata, "error out"=w752:errorcluster)  [unwired: 1 in, 2 out]
                      }
                      frame "Blackman-Harris" {
                        n113 = xnode "Spectral Measurements"("Signals"=w768, "error in (no error)"=w769) -> ("FFT - (Peak)"=w766:dynamicdata, "error out"=w767:errorcluster)  [unwired: 1 in, 2 out]
                      }
                      frame "Exact Blackman" {
                        n114 = xnode "Spectral Measurements"("Signals"=w783, "error in (no error)"=w784) -> ("FFT - (Peak)"=w781:dynamicdata, "error out"=w782:errorcluster)  [unwired: 1 in, 2 out]
                      }
                      frame "Blackman" {
                        n115 = xnode "Spectral Measurements"("Signals"=w798, "error in (no error)"=w799) -> ("FFT - (Peak)"=w796:dynamicdata, "error out"=w797:errorcluster)  [unwired: 1 in, 2 out]
                      }
                      frame "Flat Top" {
                        n116 = xnode "Spectral Measurements"("Signals"=w813, "error in (no error)"=w814) -> ("FFT - (Peak)"=w811:dynamicdata, "error out"=w812:errorcluster)  [unwired: 1 in, 2 out]
                      }
                      frame "4 Term B-Harris" {
                        n117 = xnode "Spectral Measurements"("Signals"=w828, "error in (no error)"=w829) -> ("FFT - (Peak)"=w826:dynamicdata, "error out"=w827:errorcluster)  [unwired: 1 in, 2 out]
                      }
                      frame "7 Term B-Harris" {
                        n118 = xnode "Spectral Measurements"("Signals"=w843, "error in (no error)"=w844) -> ("FFT - (Peak)"=w841:dynamicdata, "error out"=w842:errorcluster)  [unwired: 1 in, 2 out]
                      }
                      frame "Low Sidelobe" {
                        n119 = xnode "Spectral Measurements"("Signals"=w858, "error in (no error)"=w859) -> ("FFT - (Peak)"=w856:dynamicdata, "error out"=w857:errorcluster)  [unwired: 1 in, 2 out]
                      }
                    }
                  }
                  frame "Peak hold" {
                    n120 = case shown="\"Blackman\"" w875 {
                      tunnel: w874 -> [w879 w894 w909 w924 w939 w954 w969 w984 w999 w1014]
                      tunnel: w873 -> [w878 w893 w908 w923 w938 w953 w968 w983 w998 w1013]
                      tunnel: [w877 w892 w907 w922 w937 w952 w967 w982 w997 w1012] -> w872
                      tunnel: [w876 w891 w906 w921 w936 w951 w966 w981 w996 w1011] -> w871
                      frame "None", Default {
                        n121 = xnode "Spectral Measurements"("Signals"=w878, "error in (no error)"=w879) -> ("FFT - (Peak)"=w876:dynamicdata, "error out"=w877:errorcluster)  [unwired: 1 in, 2 out]
                      }
                      frame "Hanning" {
                        n122 = xnode "Spectral Measurements"("Signals"=w893, "error in (no error)"=w894) -> ("FFT - (Peak)"=w891:dynamicdata, "error out"=w892:errorcluster)  [unwired: 1 in, 2 out]
                      }
                      frame "Hamming" {
                        n123 = xnode "Spectral Measurements"("Signals"=w908, "error in (no error)"=w909) -> ("FFT - (Peak)"=w906:dynamicdata, "error out"=w907:errorcluster)  [unwired: 1 in, 2 out]
                      }
                      frame "Blackman-Harris" {
                        n124 = xnode "Spectral Measurements"("Signals"=w923, "error in (no error)"=w924) -> ("FFT - (Peak)"=w921:dynamicdata, "error out"=w922:errorcluster)  [unwired: 1 in, 2 out]
                      }
                      frame "Exact Blackman" {
                        n125 = xnode "Spectral Measurements"("Signals"=w938, "error in (no error)"=w939) -> ("FFT - (Peak)"=w936:dynamicdata, "error out"=w937:errorcluster)  [unwired: 1 in, 2 out]
                      }
                      frame "Blackman" {
                        n126 = xnode "Spectral Measurements"("Signals"=w953, "error in (no error)"=w954) -> ("FFT - (Peak)"=w951:dynamicdata, "error out"=w952:errorcluster)  [unwired: 1 in, 2 out]
                      }
                      frame "Flat Top" {
                        n127 = xnode "Spectral Measurements"("Signals"=w968, "error in (no error)"=w969) -> ("FFT - (Peak)"=w966:dynamicdata, "error out"=w967:errorcluster)  [unwired: 1 in, 2 out]
                      }
                      frame "4 Term B-Harris" {
                        n128 = xnode "Spectral Measurements"("Signals"=w983, "error in (no error)"=w984) -> ("FFT - (Peak)"=w981:dynamicdata, "error out"=w982:errorcluster)  [unwired: 1 in, 2 out]
                      }
                      frame "7 Term B-Harris" {
                        n129 = xnode "Spectral Measurements"("Signals"=w998, "error in (no error)"=w999) -> ("FFT - (Peak)"=w996:dynamicdata, "error out"=w997:errorcluster)  [unwired: 1 in, 2 out]
                      }
                      frame "Low Sidelobe" {
                        n130 = xnode "Spectral Measurements"("Signals"=w1013, "error in (no error)"=w1014) -> ("FFT - (Peak)"=w1011:dynamicdata, "error out"=w1012:errorcluster)  [unwired: 1 in, 2 out]
                      }
                    }
                  }
                }
              }
              frame "Power spectrum" {
                n131 = case shown="\"None\", Default" w1031 {
                  tunnel: w1030 -> [w1036 w1171 w1316]
                  tunnel: w1029 -> [w1035 w1170 w1315]
                  tunnel: w1028 -> [w1034 w1169 w1314]
                  tunnel: [w1033 w1168 w1313] -> w1027
                  tunnel: [w1032 w1167 w1312] -> w1026
                  frame "None", Default {
                    n132 = case shown="\"Flat Top\"" w1036 {
                      tunnel: w1035 -> [w1040 w1053 w1066 w1079 w1092 w1105 w1118 w1131 w1144 w1157]
                      tunnel: w1034 -> [w1039 w1052 w1065 w1078 w1091 w1104 w1117 w1130 w1143 w1156]
                      tunnel: [w1038 w1051 w1064 w1077 w1090 w1103 w1116 w1129 w1142 w1155] -> w1033
                      tunnel: [w1037 w1050 w1063 w1076 w1089 w1102 w1115 w1128 w1141 w1154] -> w1032
                      frame "None", Default {
                        n133 = xnode "Spectral Measurements"("Signals"=w1039, "error in (no error)"=w1040) -> ("Power Spectrum"=w1037:dynamicdata, "error out"=w1038:errorcluster)
                      }
                      frame "Hanning" {
                        n134 = xnode "Spectral Measurements"("Signals"=w1052, "error in (no error)"=w1053) -> ("Power Spectrum"=w1050:dynamicdata, "error out"=w1051:errorcluster)
                      }
                      frame "Hamming" {
                        n135 = xnode "Spectral Measurements"("Signals"=w1065, "error in (no error)"=w1066) -> ("Power Spectrum"=w1063:dynamicdata, "error out"=w1064:errorcluster)
                      }
                      frame "Blackman-Harris" {
                        n136 = xnode "Spectral Measurements"("Signals"=w1078, "error in (no error)"=w1079) -> ("Power Spectrum"=w1076:dynamicdata, "error out"=w1077:errorcluster)
                      }
                      frame "Exact Blackman" {
                        n137 = xnode "Spectral Measurements"("Signals"=w1091, "error in (no error)"=w1092) -> ("Power Spectrum"=w1089:dynamicdata, "error out"=w1090:errorcluster)
                      }
                      frame "Blackman" {
                        n138 = xnode "Spectral Measurements"("Signals"=w1104, "error in (no error)"=w1105) -> ("Power Spectrum"=w1102:dynamicdata, "error out"=w1103:errorcluster)
                      }
                      frame "Flat Top" {
                        n139 = xnode "Spectral Measurements"("Signals"=w1117, "error in (no error)"=w1118) -> ("Power Spectrum"=w1115:dynamicdata, "error out"=w1116:errorcluster)
                      }
                      frame "4 Term B-Harris" {
                        n140 = xnode "Spectral Measurements"("Signals"=w1130, "error in (no error)"=w1131) -> ("Power Spectrum"=w1128:dynamicdata, "error out"=w1129:errorcluster)
                      }
                      frame "7 Term B-Harris" {
                        n141 = xnode "Spectral Measurements"("Signals"=w1143, "error in (no error)"=w1144) -> ("Power Spectrum"=w1141:dynamicdata, "error out"=w1142:errorcluster)
                      }
                      frame "Low Sidelobe" {
                        n142 = xnode "Spectral Measurements"("Signals"=w1156, "error in (no error)"=w1157) -> ("Power Spectrum"=w1154:dynamicdata, "error out"=w1155:errorcluster)
                      }
                    }
                  }
                  frame "RMS" {
                    n143 = case shown="\"Exact Blackman\"" w1171 {
                      tunnel: w1170 -> [w1175 w1189 w1203 w1217 w1231 w1245 w1259 w1273 w1287 w1301]
                      tunnel: w1169 -> [w1174 w1188 w1202 w1216 w1230 w1244 w1258 w1272 w1286 w1300]
                      tunnel: [w1173 w1187 w1201 w1215 w1229 w1243 w1257 w1271 w1285 w1299] -> w1168
                      tunnel: [w1172 w1186 w1200 w1214 w1228 w1242 w1256 w1270 w1284 w1298] -> w1167
                      frame "None", Default {
                        n144 = xnode "Spectral Measurements"("Signals"=w1174, "error in (no error)"=w1175) -> ("Power Spectrum"=w1172:dynamicdata, "error out"=w1173:errorcluster)  [unwired: 1 in, 1 out]
                      }
                      frame "Hanning" {
                        n145 = xnode "Spectral Measurements"("Signals"=w1188, "error in (no error)"=w1189) -> ("Power Spectrum"=w1186:dynamicdata, "error out"=w1187:errorcluster)  [unwired: 1 in, 1 out]
                      }
                      frame "Hamming" {
                        n146 = xnode "Spectral Measurements"("Signals"=w1202, "error in (no error)"=w1203) -> ("Power Spectrum"=w1200:dynamicdata, "error out"=w1201:errorcluster)  [unwired: 1 in, 1 out]
                      }
                      frame "Blackman-Harris" {
                        n147 = xnode "Spectral Measurements"("Signals"=w1216, "error in (no error)"=w1217) -> ("Power Spectrum"=w1214:dynamicdata, "error out"=w1215:errorcluster)  [unwired: 1 in, 1 out]
                      }
                      frame "Exact Blackman" {
                        n148 = xnode "Spectral Measurements"("Signals"=w1230, "error in (no error)"=w1231) -> ("Power Spectrum"=w1228:dynamicdata, "error out"=w1229:errorcluster)  [unwired: 1 in, 1 out]
                      }
                      frame "Blackman" {
                        n149 = xnode "Spectral Measurements"("Signals"=w1244, "error in (no error)"=w1245) -> ("Power Spectrum"=w1242:dynamicdata, "error out"=w1243:errorcluster)  [unwired: 1 in, 1 out]
                      }
                      frame "Flat Top" {
                        n150 = xnode "Spectral Measurements"("Signals"=w1258, "error in (no error)"=w1259) -> ("Power Spectrum"=w1256:dynamicdata, "error out"=w1257:errorcluster)  [unwired: 1 in, 1 out]
                      }
                      frame "4 Term B-Harris" {
                        n151 = xnode "Spectral Measurements"("Signals"=w1272, "error in (no error)"=w1273) -> ("Power Spectrum"=w1270:dynamicdata, "error out"=w1271:errorcluster)  [unwired: 1 in, 1 out]
                      }
                      frame "7 Term B-Harris" {
                        n152 = xnode "Spectral Measurements"("Signals"=w1286, "error in (no error)"=w1287) -> ("Power Spectrum"=w1284:dynamicdata, "error out"=w1285:errorcluster)  [unwired: 1 in, 1 out]
                      }
                      frame "Low Sidelobe" {
                        n153 = xnode "Spectral Measurements"("Signals"=w1300, "error in (no error)"=w1301) -> ("Power Spectrum"=w1298:dynamicdata, "error out"=w1299:errorcluster)  [unwired: 1 in, 1 out]
                      }
                    }
                  }
                  frame "Peak hold" {
                    n154 = case shown="\"7 Term B-Harris\"" w1316 {
                      tunnel: w1315 -> [w1320 w1334 w1348 w1362 w1376 w1390 w1404 w1418 w1432 w1446]
                      tunnel: w1314 -> [w1319 w1333 w1347 w1361 w1375 w1389 w1403 w1417 w1431 w1445]
                      tunnel: [w1318 w1332 w1346 w1360 w1374 w1388 w1402 w1416 w1430 w1444] -> w1313
                      tunnel: [w1317 w1331 w1345 w1359 w1373 w1387 w1401 w1415 w1429 w1443] -> w1312
                      frame "None", Default {
                        n155 = xnode "Spectral Measurements"("Signals"=w1319, "error in (no error)"=w1320) -> ("Power Spectrum"=w1317:dynamicdata, "error out"=w1318:errorcluster)  [unwired: 1 in, 1 out]
                      }
                      frame "Hanning" {
                        n156 = xnode "Spectral Measurements"("Signals"=w1333, "error in (no error)"=w1334) -> ("Power Spectrum"=w1331:dynamicdata, "error out"=w1332:errorcluster)  [unwired: 1 in, 1 out]
                      }
                      frame "Hamming" {
                        n157 = xnode "Spectral Measurements"("Signals"=w1347, "error in (no error)"=w1348) -> ("Power Spectrum"=w1345:dynamicdata, "error out"=w1346:errorcluster)  [unwired: 1 in, 1 out]
                      }
                      frame "Blackman-Harris" {
                        n158 = xnode "Spectral Measurements"("Signals"=w1361, "error in (no error)"=w1362) -> ("Power Spectrum"=w1359:dynamicdata, "error out"=w1360:errorcluster)  [unwired: 1 in, 1 out]
                      }
                      frame "Exact Blackman" {
                        n159 = xnode "Spectral Measurements"("Signals"=w1375, "error in (no error)"=w1376) -> ("Power Spectrum"=w1373:dynamicdata, "error out"=w1374:errorcluster)  [unwired: 1 in, 1 out]
                      }
                      frame "Blackman" {
                        n160 = xnode "Spectral Measurements"("Signals"=w1389, "error in (no error)"=w1390) -> ("Power Spectrum"=w1387:dynamicdata, "error out"=w1388:errorcluster)  [unwired: 1 in, 1 out]
                      }
                      frame "Flat Top" {
                        n161 = xnode "Spectral Measurements"("Signals"=w1403, "error in (no error)"=w1404) -> ("Power Spectrum"=w1401:dynamicdata, "error out"=w1402:errorcluster)  [unwired: 1 in, 1 out]
                      }
                      frame "4 Term B-Harris" {
                        n162 = xnode "Spectral Measurements"("Signals"=w1417, "error in (no error)"=w1418) -> ("Power Spectrum"=w1415:dynamicdata, "error out"=w1416:errorcluster)  [unwired: 1 in, 1 out]
                      }
                      frame "7 Term B-Harris" {
                        n163 = xnode "Spectral Measurements"("Signals"=w1431, "error in (no error)"=w1432) -> ("Power Spectrum"=w1429:dynamicdata, "error out"=w1430:errorcluster)  [unwired: 1 in, 1 out]
                      }
                      frame "Low Sidelobe" {
                        n164 = xnode "Spectral Measurements"("Signals"=w1445, "error in (no error)"=w1446) -> ("Power Spectrum"=w1443:dynamicdata, "error out"=w1444:errorcluster)  [unwired: 1 in, 1 out]
                      }
                    }
                  }
                }
              }
              frame "Power spectral density" {
                n165 = case shown="\"RMS\"" w1462 {
                  tunnel: w1461 -> [w1467 w1602 w1747]
                  tunnel: w1460 -> [w1466 w1601 w1746]
                  tunnel: w1459 -> [w1465 w1600 w1745]
                  tunnel: [w1464 w1599 w1744] -> w1458
                  tunnel: [w1463 w1598 w1743] -> w1457
                  frame "None", Default {
                    n166 = case shown="\"None\", Default" w1467 {
                      tunnel: w1466 -> [w1471 w1484 w1497 w1510 w1523 w1536 w1549 w1562 w1575 w1588]
                      tunnel: w1465 -> [w1470 w1483 w1496 w1509 w1522 w1535 w1548 w1561 w1574 w1587]
                      tunnel: [w1469 w1482 w1495 w1508 w1521 w1534 w1547 w1560 w1573 w1586] -> w1464
                      tunnel: [w1468 w1481 w1494 w1507 w1520 w1533 w1546 w1559 w1572 w1585] -> w1463
                      frame "None", Default {
                        n167 = xnode "Spectral Measurements"("Signals"=w1470, "error in (no error)"=w1471) -> ("PSD"=w1468:dynamicdata, "error out"=w1469:errorcluster)
                      }
                      frame "Hanning" {
                        n168 = xnode "Spectral Measurements"("Signals"=w1483, "error in (no error)"=w1484) -> ("PSD"=w1481:dynamicdata, "error out"=w1482:errorcluster)
                      }
                      frame "Hamming" {
                        n169 = xnode "Spectral Measurements"("Signals"=w1496, "error in (no error)"=w1497) -> ("PSD"=w1494:dynamicdata, "error out"=w1495:errorcluster)
                      }
                      frame "Blackman-Harris" {
                        n170 = xnode "Spectral Measurements"("Signals"=w1509, "error in (no error)"=w1510) -> ("PSD"=w1507:dynamicdata, "error out"=w1508:errorcluster)
                      }
                      frame "Exact Blackman" {
                        n171 = xnode "Spectral Measurements"("Signals"=w1522, "error in (no error)"=w1523) -> ("PSD"=w1520:dynamicdata, "error out"=w1521:errorcluster)
                      }
                      frame "Blackman" {
                        n172 = xnode "Spectral Measurements"("Signals"=w1535, "error in (no error)"=w1536) -> ("PSD"=w1533:dynamicdata, "error out"=w1534:errorcluster)
                      }
                      frame "Flat Top" {
                        n173 = xnode "Spectral Measurements"("Signals"=w1548, "error in (no error)"=w1549) -> ("PSD"=w1546:dynamicdata, "error out"=w1547:errorcluster)
                      }
                      frame "4 Term B-Harris" {
                        n174 = xnode "Spectral Measurements"("Signals"=w1561, "error in (no error)"=w1562) -> ("PSD"=w1559:dynamicdata, "error out"=w1560:errorcluster)
                      }
                      frame "7 Term B-Harris" {
                        n175 = xnode "Spectral Measurements"("Signals"=w1574, "error in (no error)"=w1575) -> ("PSD"=w1572:dynamicdata, "error out"=w1573:errorcluster)
                      }
                      frame "Low Sidelobe" {
                        n176 = xnode "Spectral Measurements"("Signals"=w1587, "error in (no error)"=w1588) -> ("PSD"=w1585:dynamicdata, "error out"=w1586:errorcluster)
                      }
                    }
                  }
                  frame "RMS" {
                    n177 = case shown="\"Low Sidelobe\"" w1602 {
                      tunnel: w1601 -> [w1606 w1620 w1634 w1648 w1662 w1676 w1690 w1704 w1718 w1732]
                      tunnel: w1600 -> [w1605 w1619 w1633 w1647 w1661 w1675 w1689 w1703 w1717 w1731]
                      tunnel: [w1604 w1618 w1632 w1646 w1660 w1674 w1688 w1702 w1716 w1730] -> w1599
                      tunnel: [w1603 w1617 w1631 w1645 w1659 w1673 w1687 w1701 w1715 w1729] -> w1598
                      frame "None", Default {
                        n178 = xnode "Spectral Measurements"("Signals"=w1605, "error in (no error)"=w1606) -> ("PSD"=w1603:dynamicdata, "error out"=w1604:errorcluster)  [unwired: 1 in, 1 out]
                      }
                      frame "Hanning" {
                        n179 = xnode "Spectral Measurements"("Signals"=w1619, "error in (no error)"=w1620) -> ("PSD"=w1617:dynamicdata, "error out"=w1618:errorcluster)  [unwired: 1 in, 1 out]
                      }
                      frame "Hamming" {
                        n180 = xnode "Spectral Measurements"("Signals"=w1633, "error in (no error)"=w1634) -> ("PSD"=w1631:dynamicdata, "error out"=w1632:errorcluster)  [unwired: 1 in, 1 out]
                      }
                      frame "Blackman-Harris" {
                        n181 = xnode "Spectral Measurements"("Signals"=w1647, "error in (no error)"=w1648) -> ("PSD"=w1645:dynamicdata, "error out"=w1646:errorcluster)  [unwired: 1 in, 1 out]
                      }
                      frame "Exact Blackman" {
                        n182 = xnode "Spectral Measurements"("Signals"=w1661, "error in (no error)"=w1662) -> ("PSD"=w1659:dynamicdata, "error out"=w1660:errorcluster)  [unwired: 1 in, 1 out]
                      }
                      frame "Blackman" {
                        n183 = xnode "Spectral Measurements"("Signals"=w1675, "error in (no error)"=w1676) -> ("PSD"=w1673:dynamicdata, "error out"=w1674:errorcluster)  [unwired: 1 in, 1 out]
                      }
                      frame "Flat Top" {
                        n184 = xnode "Spectral Measurements"("Signals"=w1689, "error in (no error)"=w1690) -> ("PSD"=w1687:dynamicdata, "error out"=w1688:errorcluster)  [unwired: 1 in, 1 out]
                      }
                      frame "4 Term B-Harris" {
                        n185 = xnode "Spectral Measurements"("Signals"=w1703, "error in (no error)"=w1704) -> ("PSD"=w1701:dynamicdata, "error out"=w1702:errorcluster)  [unwired: 1 in, 1 out]
                      }
                      frame "7 Term B-Harris" {
                        n186 = xnode "Spectral Measurements"("Signals"=w1717, "error in (no error)"=w1718) -> ("PSD"=w1715:dynamicdata, "error out"=w1716:errorcluster)  [unwired: 1 in, 1 out]
                      }
                      frame "Low Sidelobe" {
                        n187 = xnode "Spectral Measurements"("Signals"=w1731, "error in (no error)"=w1732) -> ("PSD"=w1729:dynamicdata, "error out"=w1730:errorcluster)  [unwired: 1 in, 1 out]
                      }
                    }
                  }
                  frame "Peak hold" {
                    n188 = case shown="\"Low Sidelobe\"" w1747 {
                      tunnel: w1746 -> [w1751 w1765 w1779 w1793 w1807 w1821 w1835 w1849 w1863 w1877]
                      tunnel: w1745 -> [w1750 w1764 w1778 w1792 w1806 w1820 w1834 w1848 w1862 w1876]
                      tunnel: [w1749 w1763 w1777 w1791 w1805 w1819 w1833 w1847 w1861 w1875] -> w1744
                      tunnel: [w1748 w1762 w1776 w1790 w1804 w1818 w1832 w1846 w1860 w1874] -> w1743
                      frame "None", Default {
                        n189 = xnode "Spectral Measurements"("Signals"=w1750, "error in (no error)"=w1751) -> ("PSD"=w1748:dynamicdata, "error out"=w1749:errorcluster)  [unwired: 1 in, 1 out]
                      }
                      frame "Hanning" {
                        n190 = xnode "Spectral Measurements"("Signals"=w1764, "error in (no error)"=w1765) -> ("PSD"=w1762:dynamicdata, "error out"=w1763:errorcluster)  [unwired: 1 in, 1 out]
                      }
                      frame "Hamming" {
                        n191 = xnode "Spectral Measurements"("Signals"=w1778, "error in (no error)"=w1779) -> ("PSD"=w1776:dynamicdata, "error out"=w1777:errorcluster)  [unwired: 1 in, 1 out]
                      }
                      frame "Blackman-Harris" {
                        n192 = xnode "Spectral Measurements"("Signals"=w1792, "error in (no error)"=w1793) -> ("PSD"=w1790:dynamicdata, "error out"=w1791:errorcluster)  [unwired: 1 in, 1 out]
                      }
                      frame "Exact Blackman" {
                        n193 = xnode "Spectral Measurements"("Signals"=w1806, "error in (no error)"=w1807) -> ("PSD"=w1804:dynamicdata, "error out"=w1805:errorcluster)  [unwired: 1 in, 1 out]
                      }
                      frame "Blackman" {
                        n194 = xnode "Spectral Measurements"("Signals"=w1820, "error in (no error)"=w1821) -> ("PSD"=w1818:dynamicdata, "error out"=w1819:errorcluster)  [unwired: 1 in, 1 out]
                      }
                      frame "Flat Top" {
                        n195 = xnode "Spectral Measurements"("Signals"=w1834, "error in (no error)"=w1835) -> ("PSD"=w1832:dynamicdata, "error out"=w1833:errorcluster)  [unwired: 1 in, 1 out]
                      }
                      frame "4 Term B-Harris" {
                        n196 = xnode "Spectral Measurements"("Signals"=w1848, "error in (no error)"=w1849) -> ("PSD"=w1846:dynamicdata, "error out"=w1847:errorcluster)  [unwired: 1 in, 1 out]
                      }
                      frame "7 Term B-Harris" {
                        n197 = xnode "Spectral Measurements"("Signals"=w1862, "error in (no error)"=w1863) -> ("PSD"=w1860:dynamicdata, "error out"=w1861:errorcluster)  [unwired: 1 in, 1 out]
                      }
                      frame "Low Sidelobe" {
                        n198 = xnode "Spectral Measurements"("Signals"=w1876, "error in (no error)"=w1877) -> ("PSD"=w1874:dynamicdata, "error out"=w1875:errorcluster)  [unwired: 1 in, 1 out]
                      }
                    }
                  }
                }
              }
            }
          }
        }
        "FFT" <- w27
      }
    }
    n199 = Or(x=w15, y="?") -> (x .or. y?=w19:bool)
  }
  n200 = call <instrlib>:"niScope Close.vi"("instrument handle"=w3, "error in"=w5) -> ("error out"=w12:errorcluster)  [unwired: 13 in]
  n201 = call <vilib>:"Simple Error Handler.vi"("error in (no error)"=w12) -> ()  [unwired: 4 in, 5 out]
